vi "该文件同样作为子面板.vi"() -> ()   [LabVIEW 2018]
panel:
  in  "布尔":bool
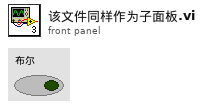
[diagram p1: front panel]
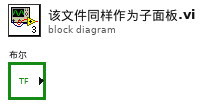
[diagram p0: block diagram]
diagram:
